vi "Check if Path Exists.vi"(8 "error in":errorcluster, 11 "File Actor in":refnum<class "File Actor.lvclass">) -> (0 "error out":errorcluster, 3 "File Actor out":refnum<class "File Actor.lvclass">)   [LabVIEW 2017, in "File Library.lvlib" / "File Actor.lvclass"]
doc: "Check to see if the specified path exists. If not, then create it."
uses:
  File Actor.lvclass
  File Actor.lvclass/File Actor.ctl
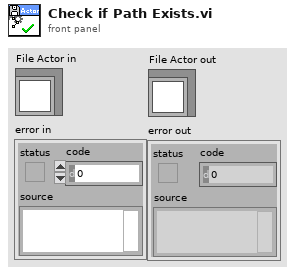
[diagram p1: front panel]
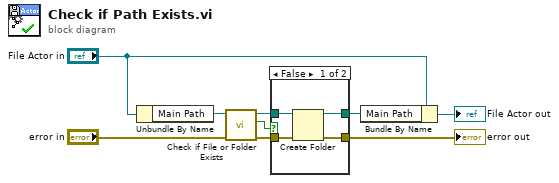
[diagram p0: block diagram]
diagram:
  n1 = Unbundle By Name("File Actor in") -> ("Main Path"=w9:path)
  n2 = call <vilib>:"Check if File or Folder Exists.vi"("error in (no error)"="error in", "path"=w9) -> ("error out"=w5:errorcluster, "file or folder exists?"=w7:bool, "dup path"=w6:path)  [unwired: 7 in]
  n3 = case shown="False" w7 {
    tunnel: w6 -> [w13 w14]
    tunnel: w5 -> [w12 w15]
    tunnel: [w11 w15] -> w4
    tunnel: [w10 w14] -> w3
    frame False {
      n4 = Create Folder(path (use dialog)=w13, error in=w12) -> (created path=w10:path, error out=w11:errorcluster)  [unwired: 1 in, 1 out]
    }
    frame True {
    }
  }
  "error out" <- w4
  n5 = Bundle By Name(cluster="File Actor in", "Main Path"=w3) -> (→"File Actor out":refnum<class "File Actor.lvclass">)
